vi "Micro-PL Stability Test v10.5.1.vi"() -> ()   [LabVIEW 2010]
uses:
  <vilib>/Utility/miscctls.llb/LVPointTypeDef.ctl
panel:
  in  "Snapshot Folder":path=path "C:/Users/WET-KORR/Desktop/Screenshots"
  in  "Camera Name":string="HD USB Camera"
  in  "Start":bool
  out "Current Time":dbl format="%<%H:%M:%S>t"
  out "Progress":u8(slide) max=10 scale=0.0..100.0
  in  "Total Unit":u16(ring)=2 caption="Unit" items=["s", "min", "h"]
  in  "Total":i32=1 min=1 max=1000 step=1
  in  "Exit":bool
  in  "Interval Unit":u16(ring)=1 caption="Unit" items=["s", "min", "h"]
  in  "Intervall":i32=1 min=0 max=1000 step=1
  # "Stability"
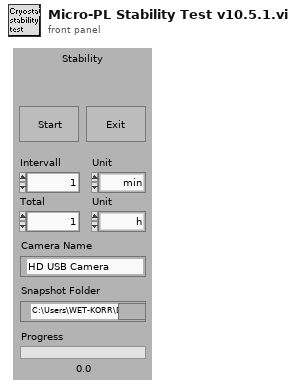
[diagram p1: front panel]
types:
  T1 = typedef "LVPointTypeDef.ctl" = cluster{"Horizontal":i16, "Vertical":i16}
  T2 = enum32{"invalid app kind", "Development System", "Run Time System", "Student Edition", "Embedded LabVIEW", "Evaluation", "Custom"}
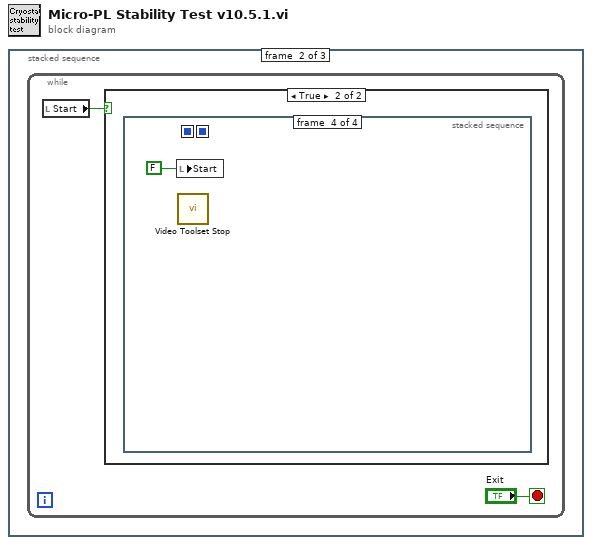
[diagram p0: block diagram]
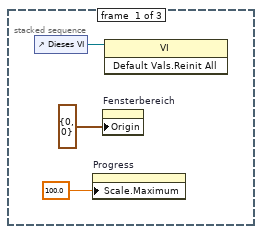
[diagram p2: hidden frame]
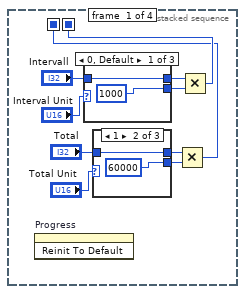
[diagram p4: hidden frame]
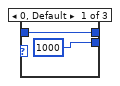
[diagram p5: hidden frame]
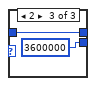
[diagram p6: hidden frame]
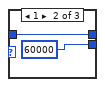
[diagram p7: hidden frame]
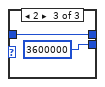
[diagram p8: hidden frame]
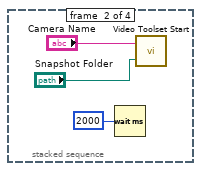
[diagram p9: hidden frame]
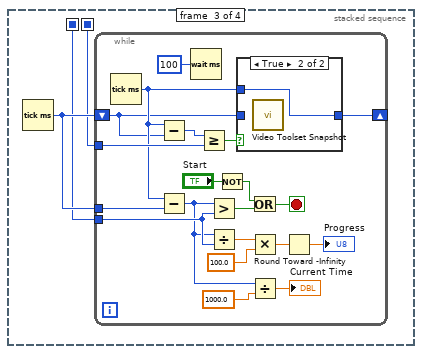
[diagram p10: hidden frame]
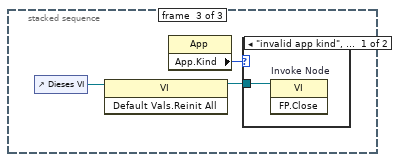
[diagram p12: hidden frame]
diagram:
  n1 = stacked-sequence {
    frame #0 {
      n2 = control-ref of="Dieses VI"() -> (w2:refnum<vi>)
      n3 = property on="Progress" class="Slide (strict)"("Scale.Maximum"=100.0 ("Skalierung.Bereich:Maximum")) -> ()  [unwired: 2 in, 2 out]
      n4 = property on="Fensterbereich" class="Pane"("Origin"=T1 {"Horizontal"=0, "Vertical"=0}) -> ()  [unwired: 2 in, 2 out]
      n5 = invoke class="VI" method="Default Vals.Reinit All"(reference=w2) -> ()  [unwired: 2 in, 3 out]
    }
    frame #1 {
      n6 = while {
        stop <- "Exit" stop-if-true
        n7 = local read "Start"() -> (w5:bool)
        n8 = case shown="True" w5 {
          frame False {
          }
          frame True {
            n9 = stacked-sequence {
              seq-local: [w7 _ _ _] -> [_ _ w32 _]
              seq-local: [w6 _ _ _] -> [_ _ w31 _]
              frame #0 {
                n10 = invoke on="Progress" class="Schieber (strikt)" method="Reinit To Default"() -> ()  [unwired: 3 in, 3 out]
                n11 = case shown="0, Default" "Interval Unit" {
                  tunnel: [1000 ("y") 60000 ("y") 3600000 ("y")] -> w15
                  tunnel: "Intervall" -> [w22 w24 w26]
                  tunnel: [w22 w24 w26] -> w12
                  frame 0, Default {
                  }
                  frame 1 {
                  }
                  frame 2 {
                  }
                }
                n12 = case shown="1" "Total Unit" {
                  tunnel: [1000 ("y") 60000 ("y") 3600000 ("y")] -> w11
                  tunnel: "Total" -> [w16 w18 w20]
                  tunnel: [w16 w18 w20] -> w10
                  frame 0, Default {
                  }
                  frame 1 {
                  }
                  frame 2 {
                  }
                }
                n13 = Multiply(x=w10, y=w11) -> (x*y=w6:i32)
                n14 = Multiply(x=w12, y=w15) -> (x*y=w7:i32)
              }
              frame #1 {
                n15 = Wait (ms)(milliseconds to wait=u32 2000 ("Timer-Wert (ms)")) -> ()  [unwired: 1 out]
                n16 = call "Video Toolset Start.vi"("Snapshot Folder"="Snapshot Folder", "Camera Name"="Camera Name") -> ()  [unwired: 1 in]
              }
              frame #2 {
                n17 = Tick Count (ms)() -> (millisecond timer value=w33:u32)
                n18 = while {
                  tunnel: w33 -> [w53]
                  shift-right: [w47] -> _
                  shift-left: w33 -> [w44]
                  tunnel: w32 -> [w49]
                  tunnel: w31 -> [w42]
                  stop <- w51 stop-if-true
                  n19 = Tick Count (ms)() -> (millisecond timer value=w45:u32)
                  n20 = Subtract(x=w45, y=w44) -> (x-y=w50:u32)
                  n21 = Subtract(x=w45, y=w53) -> (x-y=w37:u32)
                  n22 = Wait (ms)(milliseconds to wait=u32 100 ("Zu wartende ms")) -> ()  [unwired: 1 out]
                  n23 = Greater Or Equal?(x=w50, y=w49) -> (x >= y?=w48:bool)
                  n24 = Greater?(x=w37, y=w42) -> (0:w52:bool)
                  n25 = Divide(x=w37, y=w42) -> (x/y=w43:dbl)
                  n26 = Not(x="Start") -> (.not. x?=w34:bool)
                  n27 = case shown="True" w48 {
                    tunnel: [w54 w55] -> w47
                    tunnel: w44 -> [w54 _]
                    tunnel: w45 -> [_ w55]
                    frame False {
                    }
                    frame True {
                      n28 = call "Video Toolset Snapshot.vi"() -> ()  [unwired: 12 in]
                    }
                  }
                  n29 = Or(x=w34, y=w52) -> (x .or. y?=w51:bool)
                  n30 = Multiply(x=w43, y=100.0) -> (x*y=w40:dbl)
                  n31 = Divide(x=w37, y=1000.0) -> (x/y=→"Current Time":dbl)
                  n32 = Round Toward -Infinity(1:w40) -> (0:→"Progress":dbl)
                }
              }
              frame #3 {
                n33 = local write "Start"(FALSE ("Start")) -> ()
                n34 = call "Video Toolset Stop.vi"() -> ()  [unwired: 3 in]
              }
            }
          }
        }
      }
    }
    frame #2 {
      n35 = control-ref of="Dieses VI"() -> (w59:refnum<vi>)
      n36 = invoke class="VI" method="Default Vals.Reinit All"(reference=w59) -> (reference out=w57:refnum<vi>)  [unwired: 2 in, 2 out]
      n37 = property class="App"() -> ("App.Kind"=w58:T2)  [unwired: 2 in, 2 out]
      n38 = case shown="\"invalid app kind\", Default" w58 {
        tunnel: w57 -> [w60 _]
        frame "invalid app kind", Default {
          n39 = invoke on="Invoke Node" class="VI" method="FP.Close"(reference=w60) -> ()  [unwired: 2 in, 3 out]
        }
        frame "Development System" {
        }
      }
    }
  }
